vi "Configure Frequency List.vi"(6 "Enable Frequency List (Enable)":bool=TRUE, 7 "Frequency Data":dbl[](array[numeric]), 8 "error in (no error)":errorcluster, 9 "Dwell Time (1 second)":dbl=1.0, 10 "Channel (1: 1)":i32(ring)=1 items=["1"=1, "2"=2], 11 "VISA resource name":refnum<visa-resource-name>) -> (0 "error out":errorcluster, 3 "VISA resource name out":refnum<visa-resource-name>)   [LabVIEW 2016, in "Agilent 3352X Series.lvlib"]
doc: "Enable and configure the frequency List of specific channel. The settings will be stored in volatile memory and will lost when power down. \nThe frequency list controls frequency, rapidly changing to the next frequency in the list when a trigger event is received"
uses:
  Agilent 3352X Series.lvlib
  Private/Numeric Array To String(DBL).vi
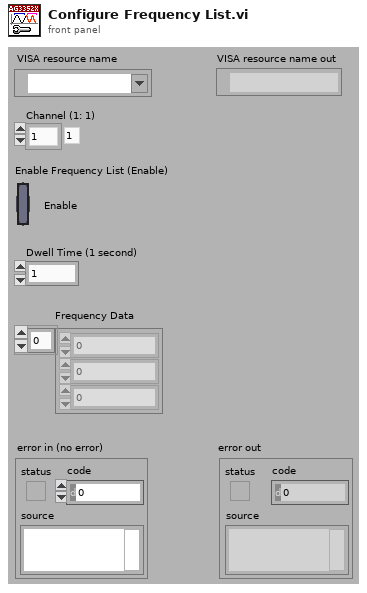
[diagram p1: front panel]
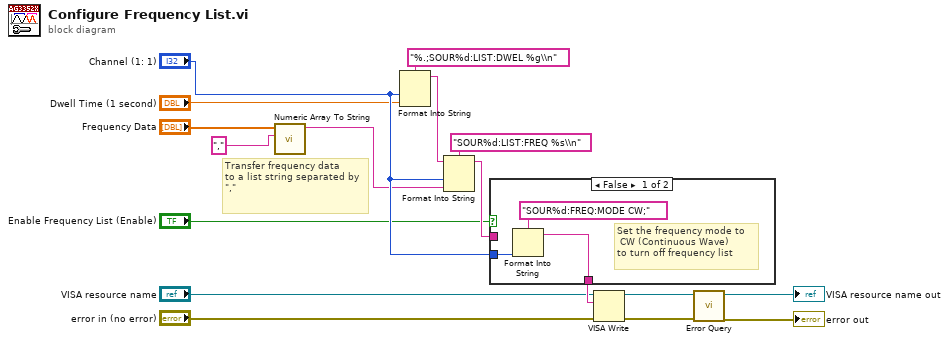
[diagram p0: block diagram]
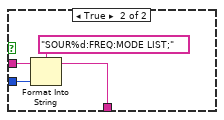
[diagram p2: hidden frame]
diagram:
  # "Transfer frequency data \nto a list string separated by \",\""
  n1 = call-poly "Numeric Array To String.vi"("Separator"="," ("Seperator"), "Numeric Array"="Frequency Data") -> ("Result String"=w2:string)  [unwired: 9 out]
  n2 = Format Into String(format string="%.;SOUR%d:LIST:DWEL %g\\n", "Channel (1: 1)", "Dwell Time (1 second)") -> (resulting string=w14:string)  [unwired: 2 in, 1 out]
  n3 = Format Into String(format string="SOUR%d:LIST:FREQ %s\\n", initial string=w14, "Channel (1: 1)", w2) -> (resulting string=w12:string)  [unwired: 1 in, 1 out]
  n4 = case shown="False" "Enable Frequency List (Enable)" {
    tunnel: "Channel (1: 1)" -> [w18 w24]
    tunnel: w12 -> [_ w22]
    tunnel: [w20 w21] -> w11
    frame False {
      # "Set the frequency mode to\n CW (Continuous Wave) \nto turn off frequency list"
      n5 = Format Into String(format string="SOUR%d:FREQ:MODE CW;", w18) -> (resulting string=w20:string)  [unwired: 2 in, 1 out]
    }
    frame True {
      n6 = Format Into String(format string="SOUR%d:FREQ:MODE LIST;", initial string=w22, w24) -> (resulting string=w21:string)  [unwired: 1 in, 1 out]
    }
  }
  n7 = VISA Write(VISA resource name="VISA resource name", write buffer=w11, error in (no error)="error in (no error)") -> (VISA resource name out=w8:refnum<visa-resource-name>, error out=w7:errorcluster)  [unwired: 1 out]
  n8 = call "Error Query.vi"("error in (no error)"=w7, "VISA resource name"=w8) -> ("error out"=→"error out":errorcluster, "VISA resource name out"=→"VISA resource name out":refnum<visa-resource-name>)  [unwired: 8 out]
